vi "ble_read_battery.vi"(6 "Connection Status":T1={"MAC Address"="", "cnx handle"=0, "cnx flags"=0, "Address Type"=125, "Connection Interval (ms)"=125, "Timeout(ms)"=125, "Latency"=0, "bonding handle"=0} {"Address Type" items=["Public", "Random"]}, 8 "error in (no error)":errorcluster, 10 "Handle table":string[][](array[string]), 11 "VISA Refnum in":refnum<visa-resource-name>) -> (0 "error out":errorcluster, 2 "battery_level(%)":u8, 3 "VISA Refnum out":refnum<visa-resource-name>)   [LabVIEW 2013]
uses:
  type_def/connection_status_bundle.ctl
  type_def/address_type.ctl
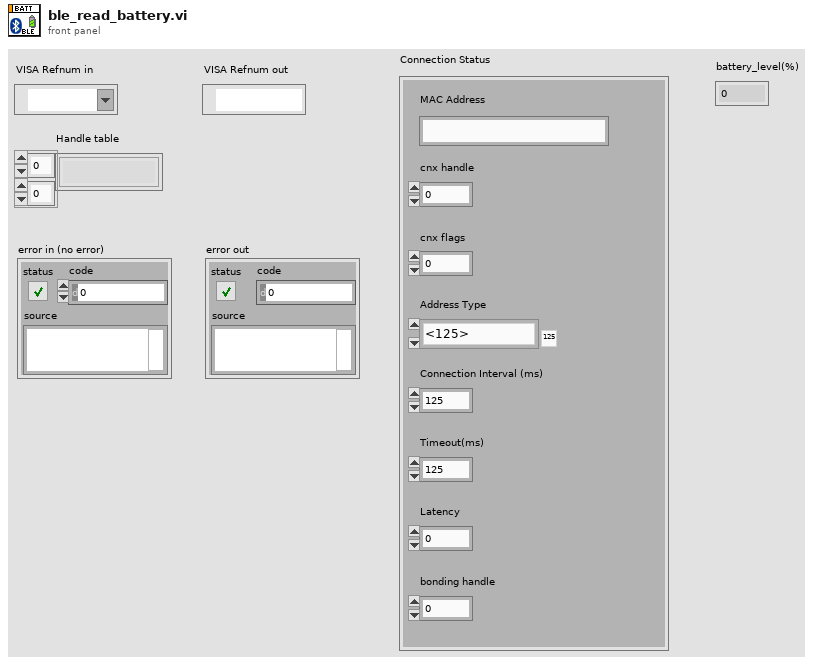
[diagram p1: front panel]
types:
  T1 = typedef "connection_status_bundle.ctl" = cluster{"MAC Address":string, "cnx handle":u8, "cnx flags":u8, "Address Type":T2, "Connection Interval (ms)":u16, "Timeout(ms)":u16, "Latency":u16, "bonding handle":u8}
  T2 = typedef "address_type.ctl" = u8
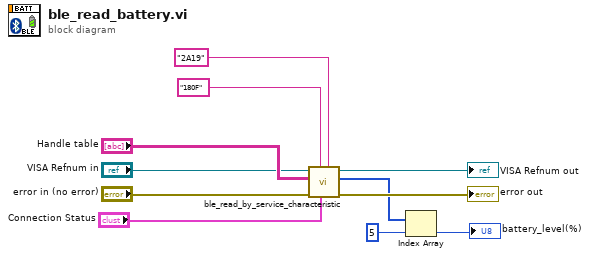
[diagram p0: block diagram]
diagram:
  n1 = call "ble_read_by_service_characteristic.vi"("Characteristic UUID"="2A19" ("MYO  UUID (16bits)"), "Connection Status"="Connection Status", "Service UUID"="180F" ("MYO  UUID (16bits)"), "error in (no error)"="error in (no error)", "Handle table"="Handle table", "COM Bluegiga in"="VISA Refnum in") -> ("error out"=→"error out":errorcluster, "characteristic value"=w3:u8[], "COM Bluegiga out"=→"VISA Refnum out":refnum<visa-resource-name>)  [unwired: 3 in]
  n2 = Index Array(array=w3, index=5) -> (element=→"battery_level(%)":u8)
